vi "Make multiple label zpl file from sn or imei list.vi"(8 "error in":errorcluster, 9 "Darkness":u32=20, 10 "Label Y offset":string="0", 11 "Label X offset":string="0") -> (0 "error out":errorcluster, 2 "Got serial number label info?":bool, 3 "zpl string for all labels":string)   [LabVIEW 2013]
panel:
  in  "ZPL PN Label file path":path
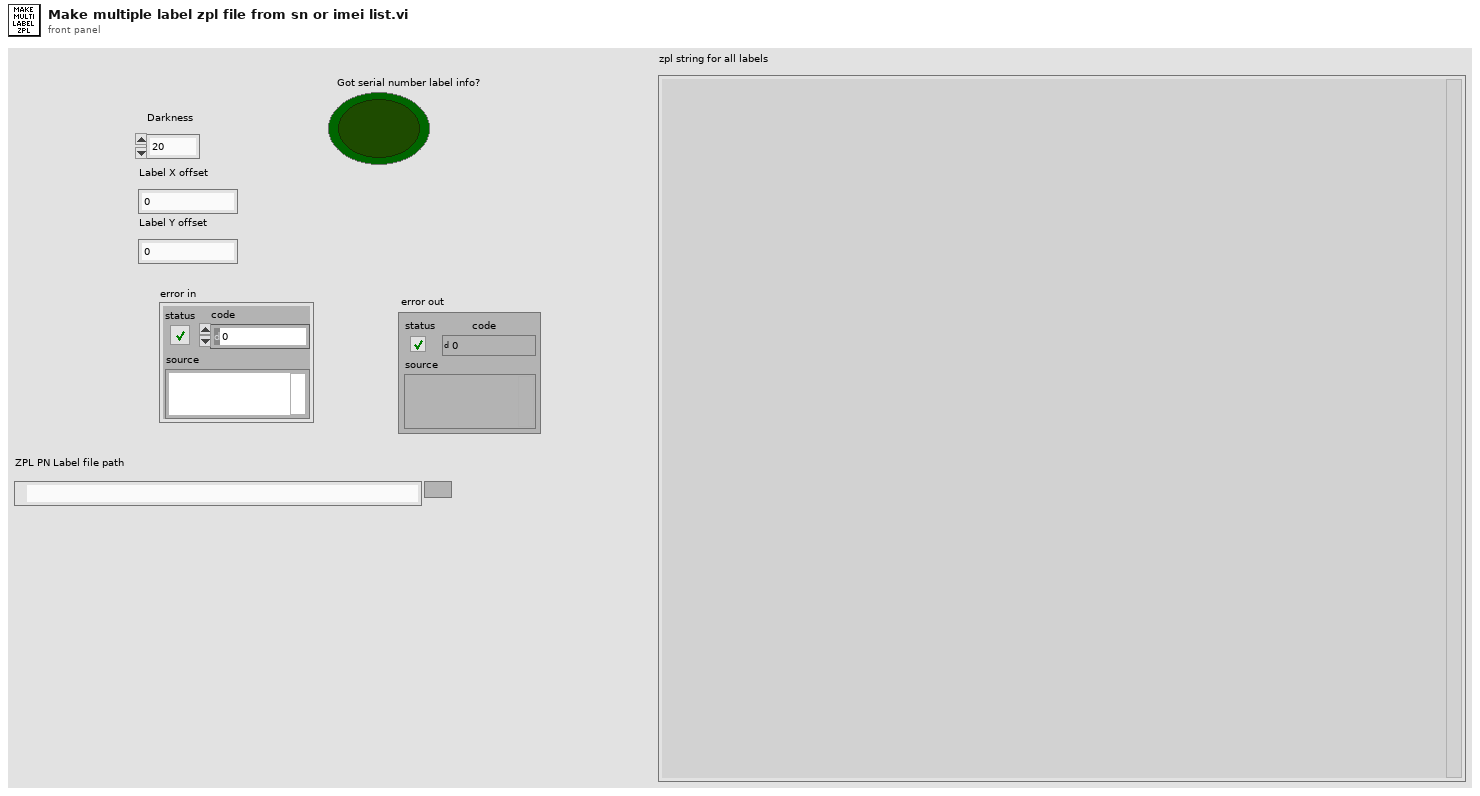
[diagram p1: front panel]
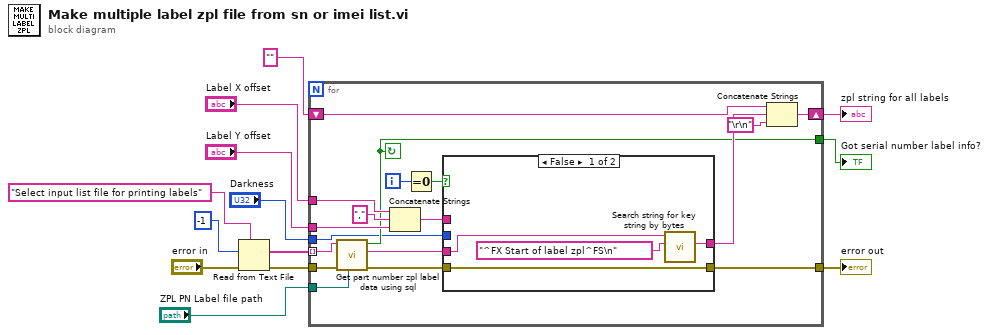
[diagram p0: block diagram]
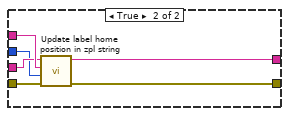
[diagram p2: hidden frame]
diagram:
  n1 = Read from Text File(prompt (Open existing file)="Select input list file for printing labels", count=-1, error in="error in") -> (text=w10:string[], error out=w9:errorcluster)  [unwired: 1 in, 2 out]
  n2 = for {
    tunnel: w10 -> [w30] mode=indexing
    tunnel: w9 -> [w31]
    shift-right: [w22] -> w6
    shift-left: "" -> [w24]
    tunnel: [w25] -> w7
    tunnel: "Label X offset" -> [w21]
    tunnel: "Label Y offset" -> [w20]
    tunnel: [w19] -> w3
    tunnel: "ZPL PN Label file path" -> [w18]
    tunnel: "Darkness" -> [w16]
    i -> [w15]
    stop <- w19 continue-if-true
    n3 = call "Get part number zpl label data using sql.vi"("ZPL PN Label file path"=w18, "error in (no error)"=w31, "Serial or IMEI"=w30) -> ("error out"=w27:errorcluster, "Label info block"=w26:string, "Got serial number label info?"=w19:bool)  [unwired: 5 in, 1 out]
    n4 = Concatenate Strings(w21, "," ("string"), w20) -> (w28:string)
    n5 = Equal To 0?(x=w15) -> (x = 0?=w14:bool)
    n6 = case shown="False" w14 {
      tunnel: w28 -> [_ w41]
      tunnel: w27 -> [w35 w40]
      tunnel: w26 -> [w34 w39]
      tunnel: [w35 w38] -> w25
      tunnel: [w32 w37] -> w23
      tunnel: w16 -> [_ w36]
      frame False {
        n7 = call "Search string for key string by bytes.vi"("Search for string"="^FX Start of label zpl^FS\n", "String"=w34) -> ("After"=w32:string)  [unwired: 5 in, 4 out]
      }
      frame True {
        n8 = call "Update label home position in zpl string.vi"("error in (no error)"=w40, "Darkness"=w36, "New label home position (x,y)"=w41, "Label ZPL"=w39) -> ("error out"=w38:errorcluster, "New Label ZPL"=w37:string)  [unwired: 6 in]
      }
    }
    n9 = Concatenate Strings(w24, w23, "\r\n") -> (w22:string)
  }
  "error out" <- w7
  "zpl string for all labels" <- w6
  "Got serial number label info?" <- w3
